vi "create Title.vi"(8 "error in (no error)":errorcluster, 11 "Chart Options":T1={"ChartName"="Chart", "BorderDashStyle"=enum."Solid", "Bordercolor"=0, "Title"={"Title"="", "TitleFontSize"=0.0, "fontName"="Arial", "font Color"=0, "Docking"=enum."Top"}, "Legend"={"Docking"=enum."None", "BorderDashStyle"=enum."Solid", "BGKcolor"=0, "BGKalpha"=103, "Title"="", "TitleSeparator"=enum."ThickLine"}} {"Legend"."BGKalpha" scale=0.0..255.0; "Title"."TitleFontSize" min=4.0 max=100.0}) -> (0 "error out":errorcluster, 3 ".NET MSChart Title":refnum<k24>)   [LabVIEW 2015, in "Graph Extensions MSChart.lvlib"]
uses:
  Graph Extensions MSChart.lvlib
  Controls/Chart.ctl
  Controls/Title.ctl
  Controls/Legend.ctl
  System.Windows.Forms.DataVisualization
  System.Drawing
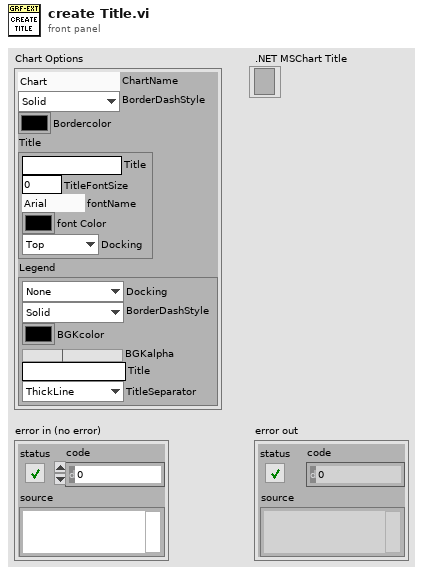
[diagram p1: front panel]
types:
  T1 = typedef "Graph Extensions MSChart.lvlib/Chart.ctl" = cluster{"ChartName":string, "BorderDashStyle":enum16{"NotSet", "Dash", "DashDot", "DashDotDot", "Dot", "Solid"}, "Bordercolor":u32, "Title":T2, "Legend":T3}
  T2 = typedef "Graph Extensions MSChart.lvlib/Title.ctl" = cluster{"Title":string, "TitleFontSize":dbl, "fontName":string, "font Color":u32, "Docking":enum16{"Top", "Right", "Bottom", "Left"}}
  T3 = typedef "Graph Extensions MSChart.lvlib/Legend.ctl" = cluster{"Docking":enum16{"None", "Top", "Right", "Bottom", "Left"}, "BorderDashStyle":enum16{"NotSet", "Dash", "DashDot", "DashDotDot", "Dot", "Solid"}, "BGKcolor":u32, "BGKalpha":u8, "Title":string, "TitleSeparator":enum16{"None", "Line", "ThickLine", "DoubleLine", "DashLine", "DotLine", "GradientLine", "ThickGradientLine"}}
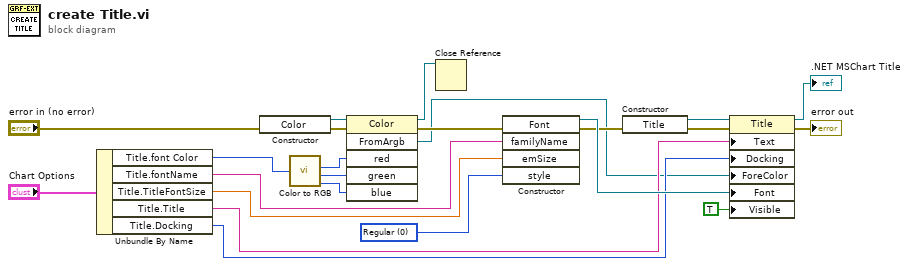
[diagram p0: block diagram]
diagram:
  w20 = 0 items=["Regular"=0, "Bold"=1, "Italic"=2, "Underline"=4, "Strikeout"=8] ("style")
  n1 = Unbundle By Name("Chart Options") -> ("Title.font Color"=w7:u32, "Title.fontName"=w6:string, "Title.TitleFontSize"=w5:dbl, "Title.Title"=w4:string, "Title.Docking"=w3:enum16{"Top", "Right", "Bottom", "Left"})
  n2 = constructor class="Color"(error in="error in (no error)") -> (reference out=w16:refnum<k24>, error out=w17:errorcluster)  [unwired: 2 in, 1 out]
  n3 = call <vilib>:"Color to RGB.vi"("Color"=w7) -> ("R"=w15:u8, "G"=w14:u8, "B"=w13:u8)  [unwired: 1 out]
  n4 = invoke class="Color" method="FromArgb"(reference=w16, error in=w17, "red"=w15, "green"=w14, "blue"=w13) -> (reference out=w1:refnum<k24>, error out=w11:errorcluster, "FromArgb"=w2:refnum<k24>)  [unwired: 1 in, 3 out]
  n5 = Close Reference(reference=w1) -> ()  [unwired: 1 in, 1 out]
  n6 = constructor class="Font"(error in=w11, "familyName"=w6, "emSize"=w5, "style"=w20) -> (reference out=w21:refnum<k24>, error out=w10:errorcluster)  [unwired: 2 in, 4 out]
  n7 = constructor class="Title"(error in=w10) -> (reference out=w19:refnum<k24>, error out=w9:errorcluster)  [unwired: 2 in, 1 out]
  n8 = property class="Title"(reference=w19, error in=w9, "Text"=w4, "Docking"=w3, "ForeColor"=w2, "Font"=w21, "Visible"=TRUE) -> (reference out=→".NET MSChart Title":refnum<k24>, error out=→"error out":errorcluster)
